vi "Generate Simulated Data.vi"(8 "error in (no error)":T2 caption="entrée d'erreur (pas d'erreur)", 11 "Type de signal":T1) -> (0 "error out":T2 caption="sortie d'erreur", 2 "Données du graphe":waveform(dbl)[](array[waveform]))   [LabVIEW 2020, in "Acquisition.lvlib"]
doc: "Génère des exemples de waveforms en fonction du type de signal dans l'entrée Configuration du matériel."
uses:
  Acquisition.lvlib
  Signal Type.ctl
  <vilib>/Analysis/NI_AALBase.lvlib
panel:
  in  "S5":bool[](array[boolean])=[FALSE, TRUE, FALSE, TRUE]
  in  "S4":bool[](array[boolean])=[FALSE, TRUE, FALSE, FALSE]
  in  "S6":bool[](array[boolean])=[FALSE, TRUE, TRUE, FALSE]
  in  "S7":bool[](array[boolean])=[FALSE, TRUE, TRUE, TRUE]
  in  "S13":bool[](array[boolean])=[TRUE, TRUE, FALSE, TRUE]
  in  "S12":bool[](array[boolean])=[TRUE, TRUE, FALSE, FALSE]
  in  "S11":bool[](array[boolean])=[TRUE, FALSE, TRUE, TRUE]
  in  "S10":bool[](array[boolean])=[TRUE, FALSE, TRUE, FALSE]
  in  "S9":bool[](array[boolean])=[TRUE, FALSE, FALSE, TRUE]
  in  "S8":bool[](array[boolean])=[TRUE, FALSE, FALSE, FALSE]
  in  "S3":bool[](array[boolean])=[TRUE, TRUE, FALSE, FALSE]
  in  "S2":bool[](array[boolean])=[FALSE, TRUE, FALSE, FALSE]
  in  "S1":bool[](array[boolean])=[TRUE, FALSE, FALSE, FALSE]
  in  "S0":bool[](array[boolean])=[FALSE, FALSE, FALSE, FALSE]
  in  "nom du périphérique":tag="Dev1"
  out "Graphe déroulant":dynamicdata(graph)
  # "ALLO MON GROS TAPON\n\nCOMPTE TES SWITCH A L'ENDROIT AVANT QUE JE TE CASSE TES KNEECAP"
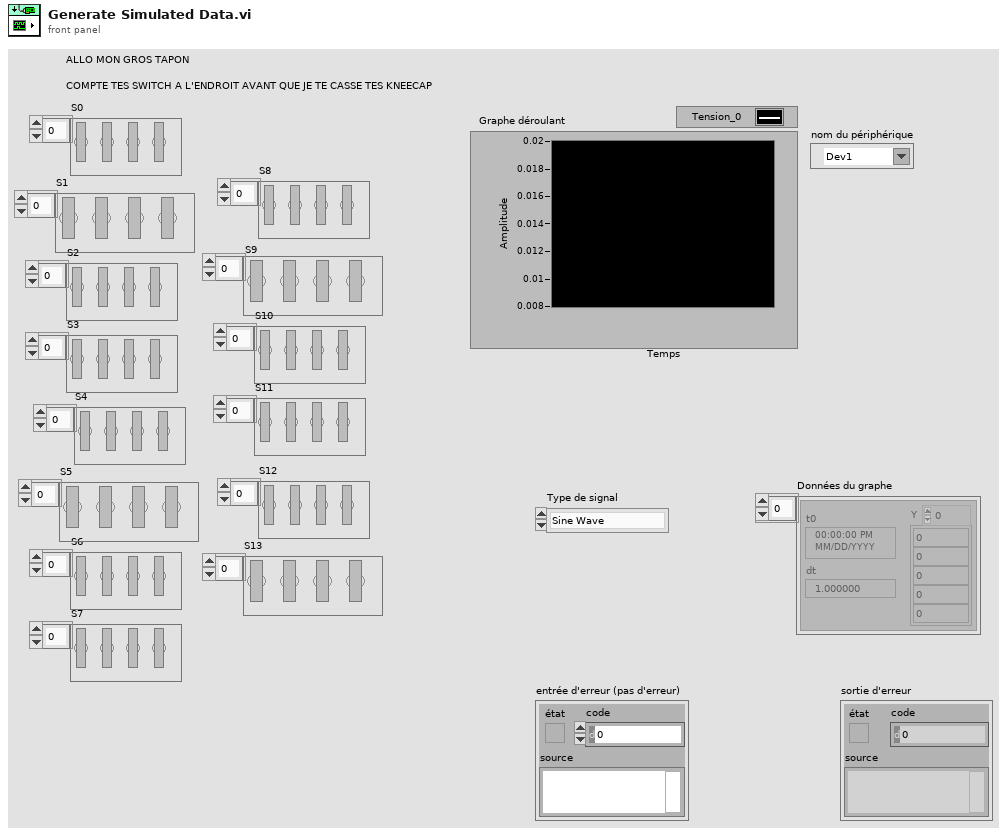
[diagram p1: front panel]
types:
  T1 = typedef "Acquisition.lvlib/Signal Type.ctl" = enum16{"Sine Wave", "Square with Noise", "Signal triangulaire", "Simulation DAQ"}
  T2 = cluster{"état":bool, "code":i32, "source":string}
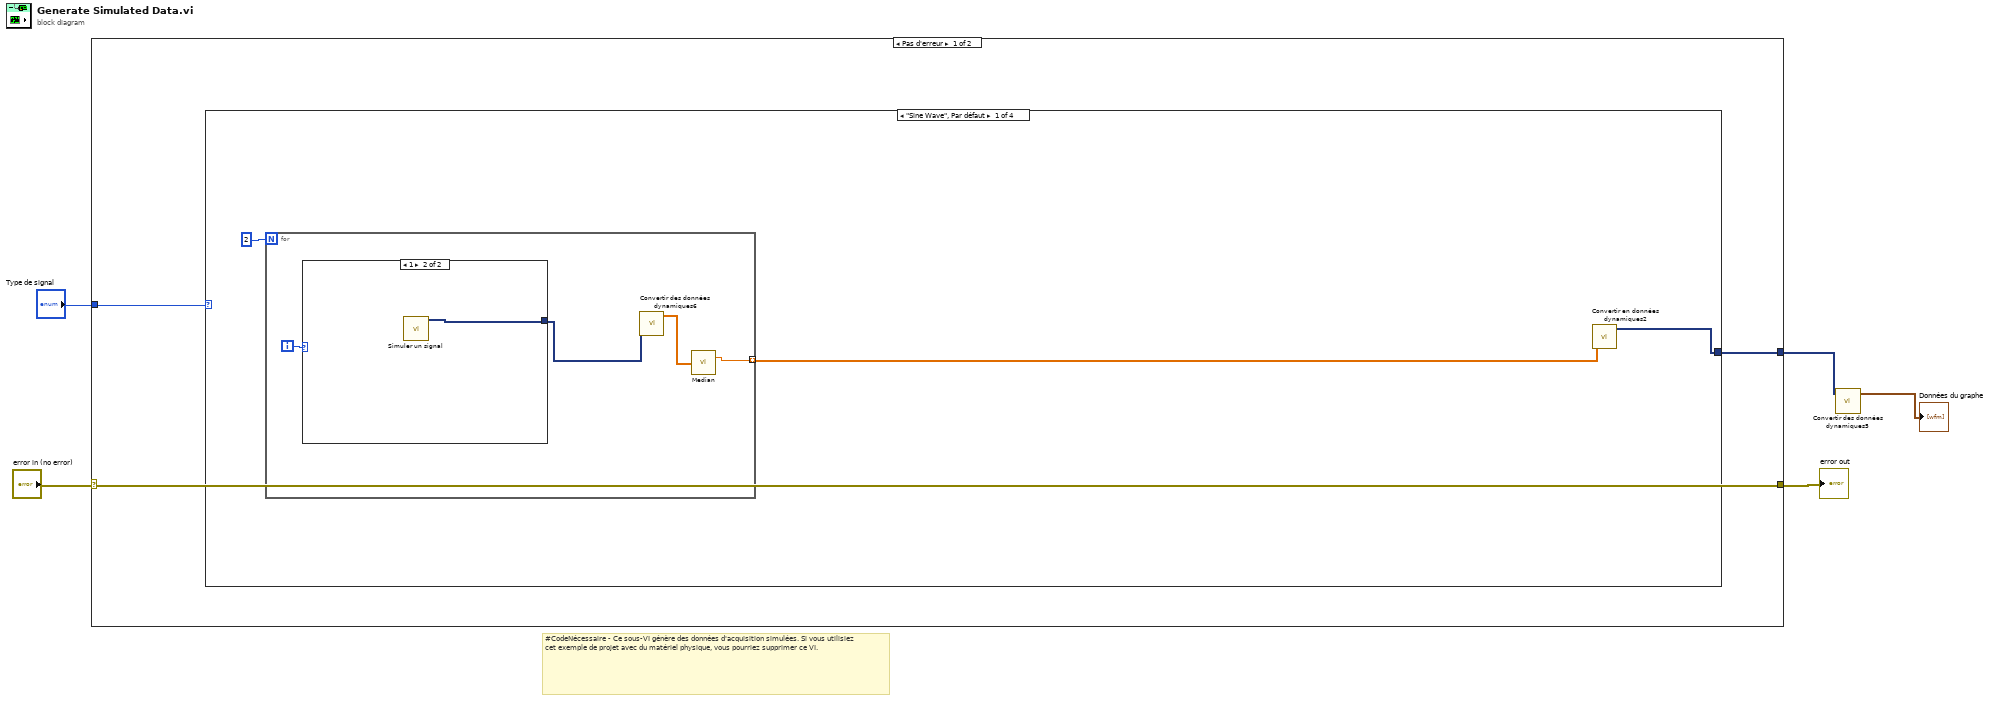
[diagram p0: block diagram]
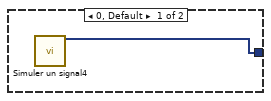
[diagram p2: hidden frame]
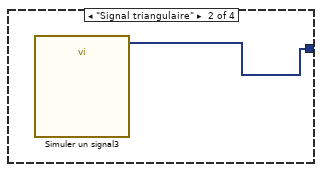
[diagram p3: hidden frame]
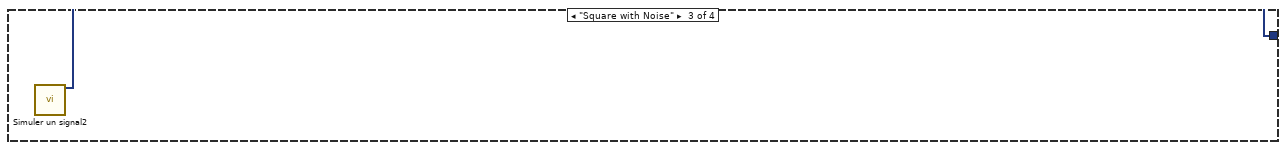
[diagram p4: hidden frame]
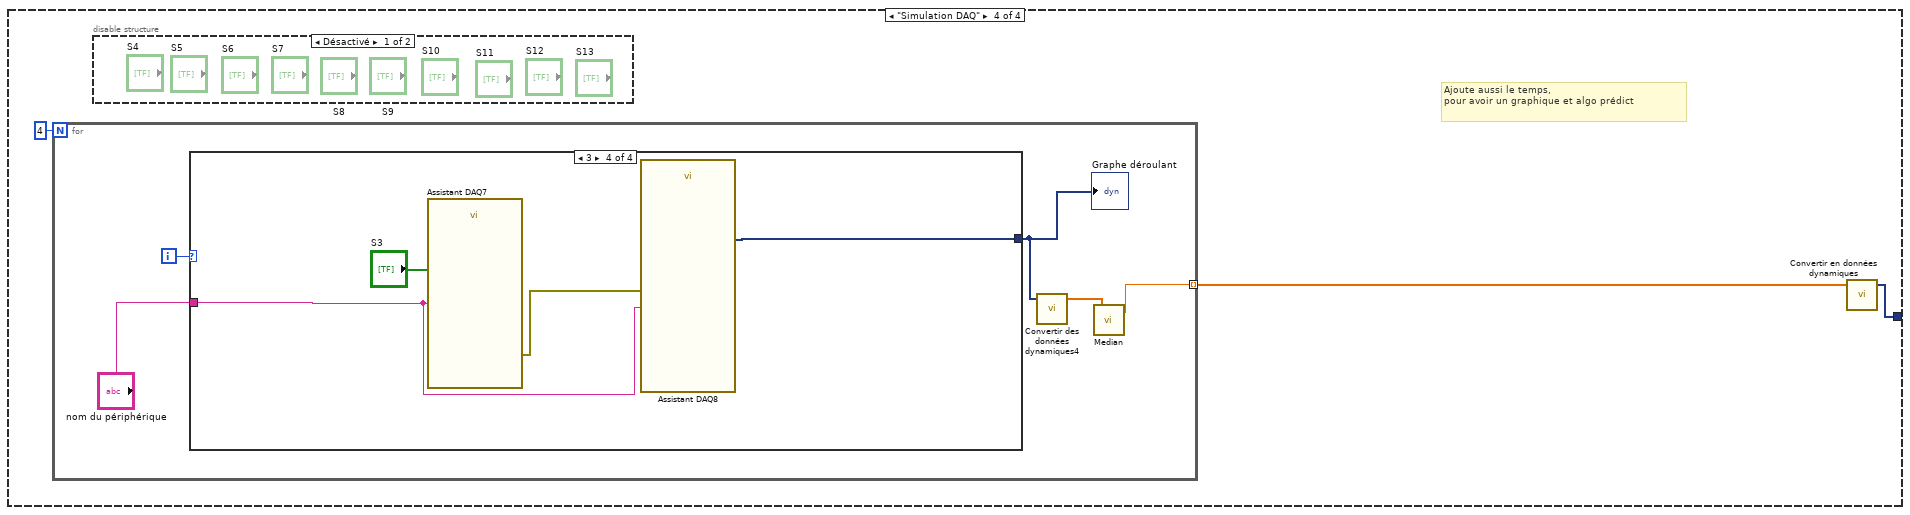
[diagram p5: hidden frame]
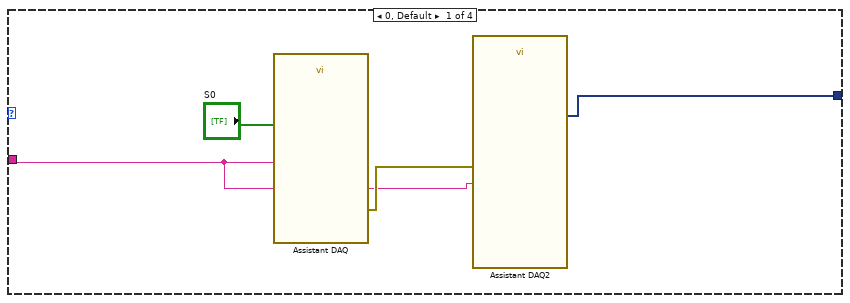
[diagram p6: hidden frame]
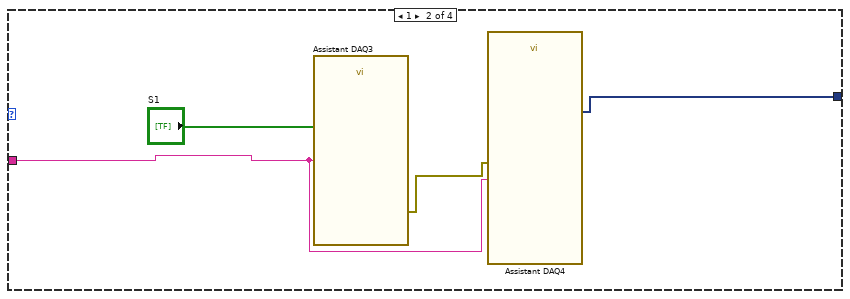
[diagram p7: hidden frame]
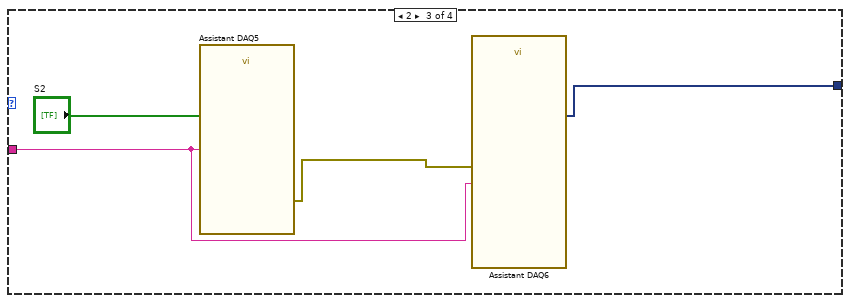
[diagram p8: hidden frame]
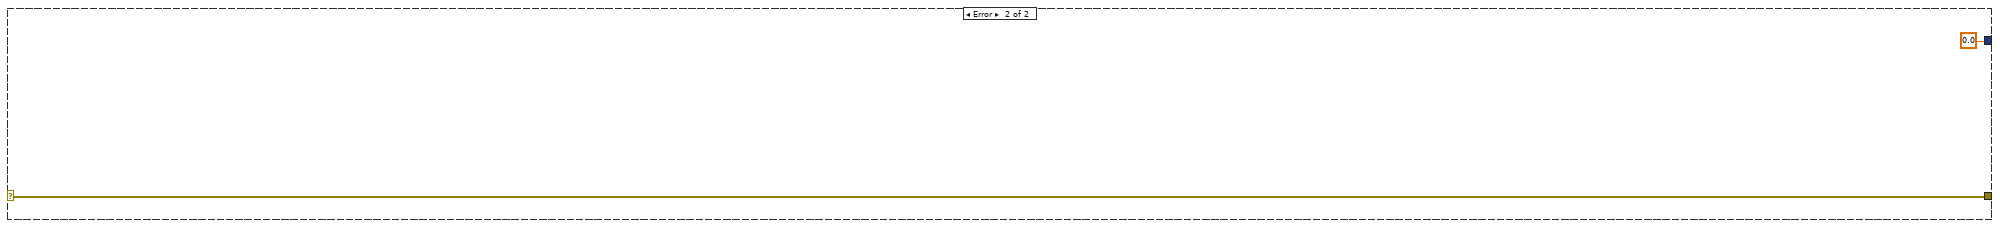
[diagram p10: hidden frame]
diagram:
  # "#CodeNécessaire - Ce sous-VI génère des données d'acquisition simulées. Si vous utilisiez cet exemple de projet avec du matériel physique, vous pourriez supprimer ce VI."
  n1 = case shown="Pas d'erreur" "error in (no error)" {
    selector: "error in (no error)" -> [w8 w45]
    tunnel: [w8 w45] -> w4
    tunnel: "Type de signal" -> [w7 _]
    tunnel: [w6 0.0] -> w1
    frame No Error {
      n2 = case shown="\"Sine Wave\", Par défaut" w7 {
        tunnel: [w9 w18 w19 w21] -> w6
        frame "Sine Wave", Default {
          n3 = for {
            N: 2 -> [_]
            tunnel: [w12] -> w10 mode=indexing
            i -> [w15]
            n4 = case shown="1" w15 {
              tunnel: [w16 w17] -> w14
              frame 0, Default {
                n5 = call "Simuler un signal4"() -> ("CC"=w16:dynamicdata)  [unwired: 14 in, 1 out]
              }
              frame 1 {
                n6 = call "Simuler un signal"() -> ("Sinus avec Bruit uniforme"=w17:dynamicdata)  [unwired: 14 in, 1 out]
              }
            }
            n7 = call "Convertir des données dynamiques6"("Dynamic Data Type"=w14) -> ("Array"=w13:dbl[])  [unwired: 3 in]
            n8 = call <vilib>:"Median.vi"("X"=w13) -> ("median"=w12:dbl)  [unwired: 1 out]
          }
          n9 = call "Convertir en données dynamiques2"("Array"=w10) -> ("Dynamic Data Type"=w9:dynamicdata)  [unwired: 3 in]
        }
        frame "Signal triangulaire" {
          n10 = call "Simuler un signal3"() -> ("Triangle"=w18:dynamicdata)  [unwired: 14 in, 1 out]
        }
        frame "Square with Noise" {
          n11 = call "Simuler un signal2"() -> ("Square with Gaussian Noise"=w19:dynamicdata)  [unwired: 14 in, 1 out]
        }
        frame "Simulation DAQ" {
          # "Ajoute aussi le temps,\npour avoir un graphique et algo prédict"
          n12 = for {
            N: 4 -> [_]
            tunnel: [w26] -> w20 mode=indexing
            i -> [w27]
            n13 = case shown="3" w27 {
              tunnel: "nom du périphérique" -> [w30 w33 w37 w41]
              tunnel: [w29 w32 w36 w42] -> w25
              frame 0, Default {
                n14 = call "Assistant DAQ"("data"="S0", "nom du périphérique"=w30) -> ("error out"=w31:errorcluster)  [unwired: 16 in, 1 out]
                n15 = call "Assistant DAQ2"("error in"=w31, "nom du périphérique"=w30) -> ("data"=w29:dynamicdata)  [unwired: 15 in, 2 out]
              }
              frame 1 {
                n16 = call "Assistant DAQ3"("data"="S1", "nom du périphérique"=w33) -> ("error out"=w34:errorcluster)  [unwired: 16 in, 1 out]
                n17 = call "Assistant DAQ4"("error in"=w34, "nom du périphérique"=w33) -> ("data"=w32:dynamicdata)  [unwired: 15 in, 2 out]
              }
              frame 2 {
                n18 = call "Assistant DAQ5"("data"="S2", "nom du périphérique"=w37) -> ("error out"=w38:errorcluster)  [unwired: 16 in, 1 out]
                n19 = call "Assistant DAQ6"("error in"=w38, "nom du périphérique"=w37) -> ("data"=w36:dynamicdata)  [unwired: 15 in, 2 out]
              }
              frame 3 {
                n20 = call "Assistant DAQ7"("data"="S3", "nom du périphérique"=w41) -> ("error out"=w40:errorcluster)  [unwired: 16 in, 1 out]
                n21 = call "Assistant DAQ8"("error in"=w40, "nom du périphérique"=w41) -> ("data"=w42:dynamicdata)  [unwired: 15 in, 2 out]
              }
            }
            "Graphe déroulant" <- w25
            n22 = call "Convertir des données dynamiques4"("Dynamic Data Type"=w25) -> ("Array"=w24:dbl[])  [unwired: 3 in]
            n23 = call <vilib>:"Median.vi"("X"=w24) -> ("median"=w26:dbl)  [unwired: 1 out]
          }
          n24 = disable-structure shown="Désactivé" {
            frame Disabled {
            }
            frame Enabled {
            }
          }
          n25 = call "Convertir en données dynamiques"("Array"=w20) -> ("Dynamic Data Type"=w21:dynamicdata)  [unwired: 3 in]
        }
      }
    }
    frame Error {
    }
  }
  "error out" <- w4
  n26 = call "Convertir des données dynamiques5"("Dynamic Data Type"=w1) -> ("Array of Waveform"=→"Données du graphe":waveform(dbl)[])  [unwired: 3 in]
